vi "variant array to numeric array.vi"(8 "error in (no error)":errorcluster, 10 "Datatype":T1, 11 "variant":variant) -> (0 "error out":errorcluster, 3 "Array":dbl[](array[numeric]))   [LabVIEW 2020]
uses:
  Datatype--enum.ctl
  DS_variant_array.lvclass
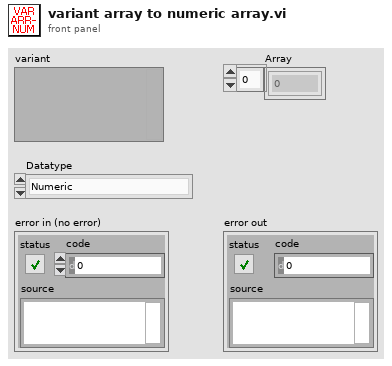
[diagram p1: front panel]
types:
  T1 = typedef "DS_variant_array.lvclass/Datatype--enum.ctl" = enum16{"Numeric", "String"}
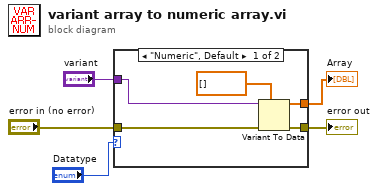
[diagram p0: block diagram]
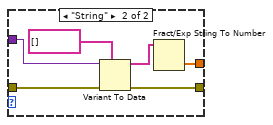
[diagram p2: hidden frame]
diagram:
  n1 = case shown="\"Numeric\", Default" "Datatype" {
    tunnel: "variant" -> [w9 w15]
    tunnel: "error in (no error)" -> [w8 w11]
    tunnel: [w7 w12] -> w5
    tunnel: [w6 w13] -> w4
    frame "Numeric", Default {
      n2 = Variant To Data(error in=w8, type=dbl[] [], Variant=w9) -> (data=w6:dbl[], error out=w7:errorcluster)
    }
    frame "String" {
      n3 = Variant To Data(error in=w11, type=string[] [], Variant=w15) -> (data=w16:string[], error out=w12:errorcluster)
      n4 = Fract/Exp String To Number(string=w16) -> (number=w13:dbl[])  [unwired: 3 in, 1 out]
    }
  }
  "error out" <- w5
  "Array" <- w4
